vi "Z900_navX_Internal_ProcessingLoop.vi"(11 "navX Device":T2={"Interface"={"Protocol"=enum."SERIAL", "Update Rate (4Hz-100Hz)"=4, "navX Open TypeDef"=variant}, "Notify Packet"=refnum, "Loop VI Refnum"=refnum, "Ready to Close Occurrence Refnum"=refnum} {"Interface"."Update Rate (4Hz-100Hz)" min=4 max=60 step=1}) -> (0 "error out":errorcluster)   [LabVIEW 2015, in "navX Library v2.lvlib"]
doc: "This navX VI handles the reading/writing for the navX. All of the good stuff is in here.\nTHIS VI SHOULD NOT BE CALLED BY THE USER!"
uses:
  navX Library v2.lvlib
  _TypeDefs/Z900_navX_DeviceTypeDef.ctl
  _TypeDefs/Z900_navX_ProtocolTypeDef.ctl
  _TypeDefs/Z900_navX_NotifyPacketTypeDef.ctl
  _TypeDefs/Z900_navX_ActionTypeDef.ctl
  _TypeDefs/Z900_navX_DeviceProcessingLoopStatus.ctl
  <vilib>/Platform/TimedLoop/XDataNode/timing_clust.ctl
  <vilib>/Platform/TimedLoop/XDataNode/nitl_modes.ctl
  <vilib>/Platform/TimedLoop/XDataNode/wakeup.ctl
  _TypeDefs/Z900_navX_InternalTimoutStatusTypeDef.ctl
  SERIAL/Z900_navX_SERIAL_PacketChecksum.vi
  SERIAL/Z900_navX_SERIAL_CapturePacket.vi
  SERIAL/Z900_navX_SERIAL_DecodePacket.vi
  _Util/Decode Protocol/Z900_navX_Util_DecodeProtocol_UInt16.vi
  SERIAL/Z900_navX_SERIAL_ValidatePacketChecksum.vi
  SERIAL/Z900_navX_SERIAL_ValidatePacketTermination.vi
  _Util/Encode Protocol/Z900_navX_Util_EncodeProtocol_SignedHundredths.vi
  _Util/Encode Protocol/Z900_navX_Util_EncodeProtocol_UnsignedHundredths.vi
  _Util/Encode Protocol/Z900_navX_Util_EncodeProtocol_UInt16.vi
  _Util/Z900_navX_Util_LittleEndian_to_BigEndian.vi
  _Util/Encode Protocol/Z900_navX_Util_EncodeProtocol_Int16.vi
  _Util/Z900_navX_Util_BigEndian_to_LittleEndian.vi
  <vilib>/Rock Robotics/WPI/SPI/WPI_SPIClose.vi
  <vilib>/Rock Robotics/WPI/I2C/WPI_I2CClose.vi
  <vilib>/Rock Robotics/WPI/SerialPort/WPI_SerialPortClose.vi
  <vilib>/Rock Robotics/WPI/SerialPort/WPI_SerialPortReset.vi
  <vilib>/Rock Robotics/SystemInterfaces/Utilities/FPGA_UtilitiesRead LocalTime.vi
  <vilib>/Utility/error.llb/Error Cluster From Error Code.vi
  SPI/Z900_navX_SPI_CRC.vi
  <vilib>/Rock Robotics/WPI/SPI/WPI_SPIRead.vi
  <vilib>/Rock Robotics/WPI/SPI/WPI_SPIWrite.vi
  <vilib>/Rock Robotics/WPI/I2C/WPI_I2CRead.vi
  <vilib>/Rock Robotics/WPI/I2C/WPI_I2CWrite.vi
  <vilib>/Rock Robotics/WPI/SerialPort/WPI_SerialPortGetBytesReceived.vi
  <vilib>/Rock Robotics/WPI/SerialPort/WPI_SerialPortRead.vi
  <vilib>/Rock Robotics/WPI/SerialPort/WPI_SerialPortFlush.vi
  <vilib>/Rock Robotics/WPI/SerialPort/WPI_SerialPortWrite.vi
  <vilib>/Rock Robotics/WPI/SPI/WPI_SPIOpen.vi
  <vilib>/Rock Robotics/WPI/I2C/WPI_I2COpen.vi
  <vilib>/Rock Robotics/WPI/SerialPort/WPI_SerialPortTermination.vi
  _NI WPI Serial USB/WPI_SerialPortOpen_USB.vi
  <vilib>/platform/TimedLoop/XDataNode/XDataNode.xnode
  <vilib>/Platform/TimedLoop/XDataNode/XDNodeRunTimeDep.lvlib
panel:
  out "Device ProcessingLoop Status":T1
  in  "Halt":bool
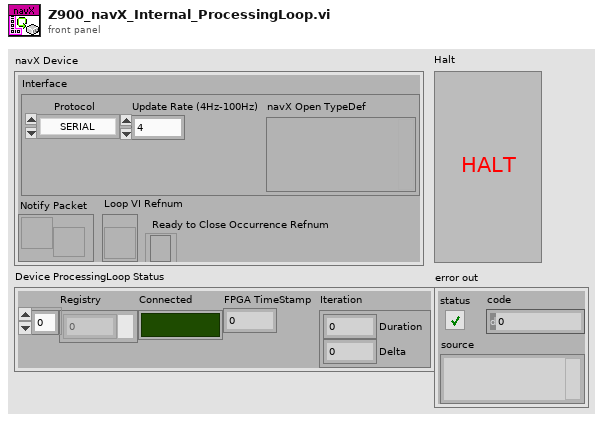
[diagram p1: front panel]
types:
  T1 = typedef "navX Library v2.lvlib/Z900_navX_DeviceProcessingLoopStatus.ctl" = cluster{"Registry":u8[], "Connected":bool, "FPGA TimeStamp":dbl, "Iteration":cluster{"Duration":i64, "Delta":i64}}
  T2 = typedef "navX Library v2.lvlib/Z900_navX_DeviceTypeDef.ctl" = cluster{"Interface":cluster{"Protocol":T3, "Update Rate (4Hz-100Hz)":u8, "navX Open TypeDef":variant}, "Notify Packet":refnum<notifier>, "Loop VI Refnum":refnum<vi>, "Ready to Close Occurrence Refnum":refnum<k4>}
  T3 = typedef "navX Library v2.lvlib/Z900_navX_ProtocolTypeDef.ctl" = enum16{"SERIAL", "I2C", "SPI"}
  T4 = typedef "navX Library v2.lvlib/Z900_navX_InternalTimoutStatusTypeDef.ctl" = cluster{"Last Valid FPGA Time":dbl, "Error Count":i32, "Initialized":bool}
  T5 = typedef "navX Library v2.lvlib/Z900_navX_InterfaceTypeDef.ctl" = cluster{"SerialPortRef":T6, "I2CDevRef":T7, "SPIDevRef":T9}
  T6 = typedef "WPI_SerialPortRef.ctl" = cluster{"DevStatus":errorcluster, "Serial Port Name":refnum<visa-resource-name>}
  T7 = typedef "WPI_I2CDevRef.ctl" = cluster{"DevStatus":errorcluster, "Device Address":u8, "Handle":i32, "I2C Bus":T8}
  T8 = typedef "i2c_bus.ctl" = enum16{"I2C On-Board", "I2C MXP", "Invalid"}
  T9 = typedef "WPI_SPIDevRef.ctl" = cluster{"DevStatus":errorcluster, "Handle":i32, "SPI Bus":T10}
  T10 = typedef "spi_bus.ctl" = enum16{"SPI On-Board, CS0", "SPI On-Board, CS1", "SPI On-Board, CS2", "SPI On-Board, CS3", "SPI MXP", "Invalid"}
  T11 = typedef "XDNodeRunTimeDep.lvlib/timing_clust.ctl" = cluster{"Expected End [f-1]":u64, "Actual End [f-1]":u64, "Finished Late? [f-1]":bool, "Expected End [i-1]":u64, "Actual End [i-1]":u64, "Finished Late? [i-1]":bool, "Expected Start [i]":u64, "Actual Start [i]":u64, "Expected Start [f]":u64, "Actual Start [f]":u64, "Source Name":string, "Structure Name":string, "Period":i64, "Deadline":i64, "Offset":i64, "Start":i64, "Priority":i32, "Timeout":i32, "Mode":T12, "Wakeup Reason":T13, "Error":errorcluster, "Source Type":string, "Secondary Source Type":string, "Global End Time":u64, "Global Start Time":u64, "Frame Duration":u64, "Iteration Duration":u64, "Assigned CPU":i32, "I/O Scan Engine Mode":u32}
  T12 = typedef "XDNodeRunTimeDep.lvlib/nitl_modes.ctl" = enum32{"No Change", "Process missed periods, maintain original phase", "Discard missed periods, maintain original phase", "Process missed periods, ignore original phase", "Discard missed periods, ignore original phase"}
  T13 = typedef "XDNodeRunTimeDep.lvlib/wakeup.ctl" = enum32{"Normal", "Aborted", "Asynchronous wakeup", "Timing source error", "Timed loop error", "Timeout"}
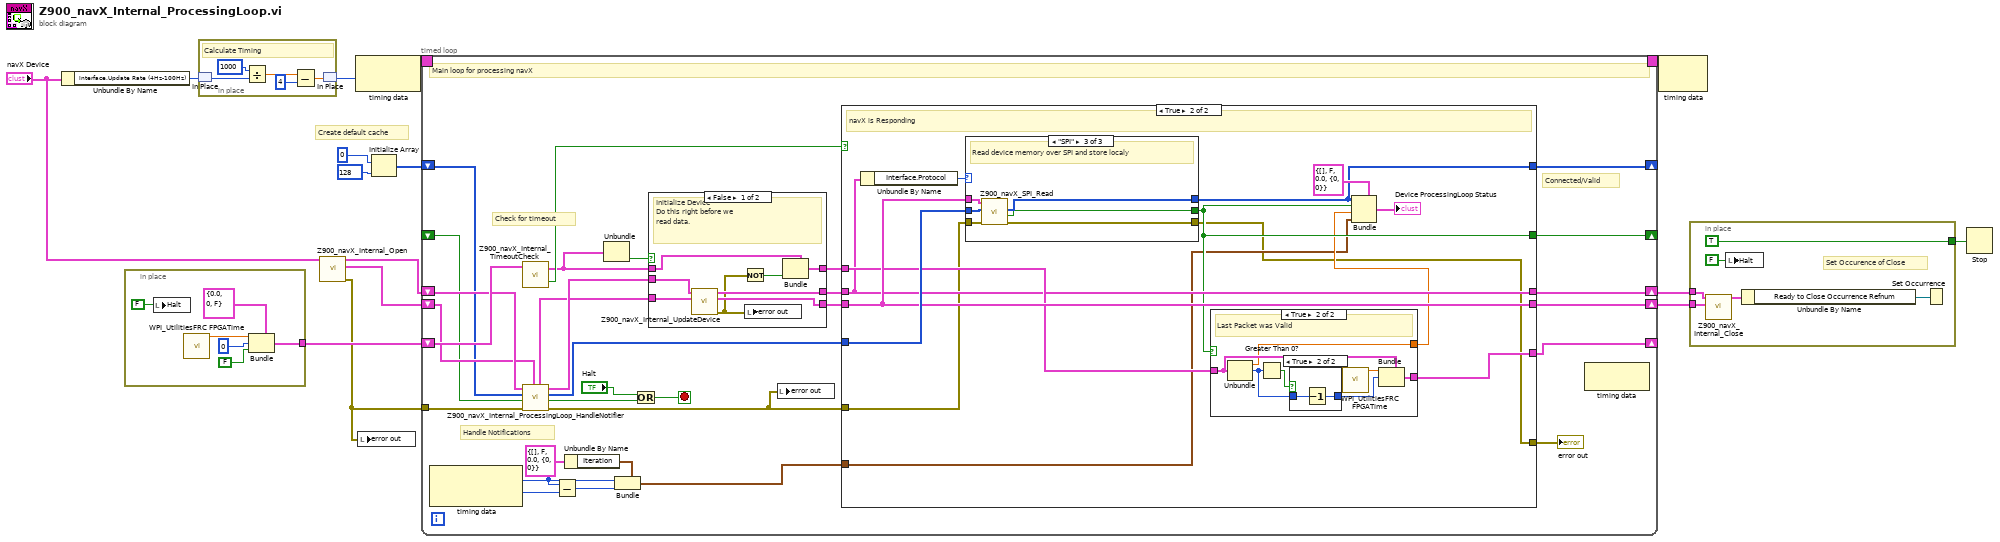
[diagram p0: block diagram]
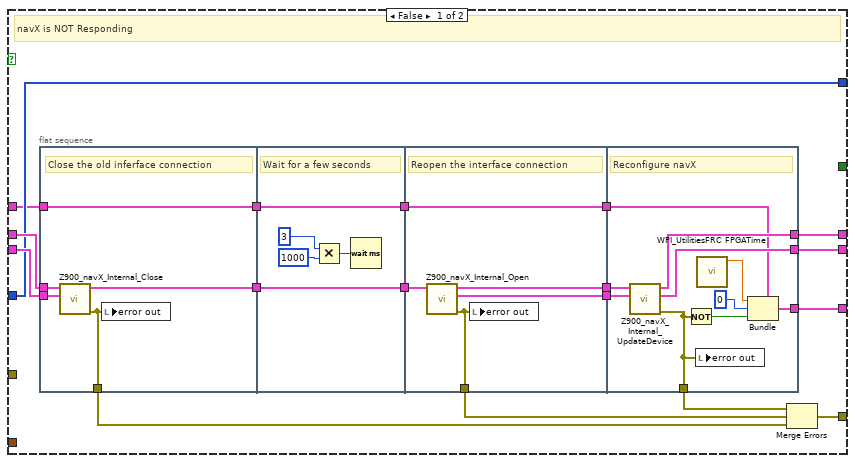
[diagram p3: hidden frame]
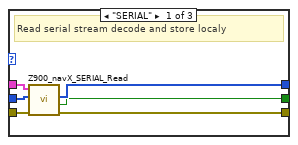
[diagram p4: hidden frame]
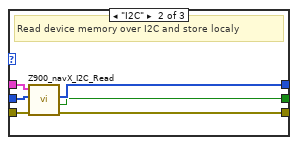
[diagram p5: hidden frame]
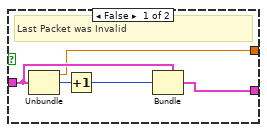
[diagram p6: hidden frame]
diagram:
  # "Create default cache"
  n1 = Unbundle By Name("navX Device") -> ("Interface.Update Rate (4Hz-100Hz)"=w12:u8)
  n2 = in-place {
    in-place-border: [w19] -> w7
    n3 = local write "Halt"(FALSE ("Halt")) -> ()
    n4 = call <vilib>:"WPI_UtilitiesFRC FPGATime.vi"() -> ("FPGA Time"=w20:dbl)  [unwired: 10 in, 1 out]
    n5 = Bundle(cluster=T4 {"Last Valid FPGA Time"=0.0, "Error Count"=0, "Initialized"=FALSE}, "Last Valid FPGA Time"=w20, "Error Count"=0, "Initialized"=FALSE) -> (w19:T4)
  }
  n6 = in-place {
    # "Calculate Timing"
    n7 = in-place-match #1(w12) -> (w25:u8)
    n8 = Divide(x=1000, y=w25) -> (x/y=w23:dbl)
    n9 = Subtract(x=w23, y=4) -> (x-y=w22:dbl)
    n10 = in-place-match #1(w22) -> (w13:u8)
  }
  n11 = call "Z900_navX_Internal_Open.vi"("navX Device"="navX Device") -> ("error out"=w1:errorcluster, "Interface TypeDefs"=w8:T5, "navX Device"=w6:T2)  [unwired: 8 in]
  n12 = node-c288(w13) -> (w15:T11)
  n13 = local write "error out"(w1) -> ()
  n14 = Initialize Array(u8 0 ("Received Data"), 128 ("hex")) -> (w11:u8[])
  n15 = timed-loop {
    timing: w15 -> [_]
    timing-out: [_] -> w14
    shift-right: [w57] -> _
    shift-left: w11 -> [w43]
    shift-right: [w54] -> w10
    shift-left: w6 -> [w45]
    shift-right: [w55] -> w9
    shift-left: w8 -> [w44]
    shift-right: [w56] -> _
    shift-left: w7 -> [w49]
    tunnel: w1 -> [w41]
    shift-right: [w46] -> _
    shift-left: _ -> [w42]
    stop <- w34 stop-if-true
    # "Check for timeout"
    # "Handle Notifications"
    # "Connected/Valid"
    # "Main loop for processing navX"
    n16 = node-c288() -> (w29:i64, w33:i64)  [unwired: 1 in]
    n17 = call "Z900_navX_Internal_TimeoutCheck.vi"("Timout Status (in)"=w49) -> ("TIMEOUT!"=w48:bool, "Timout Status (out)"=w47:T4)  [unwired: 2 in]
    n18 = call "Z900_navX_Internal_ProcessingLoop_HandleNotifier.vi"("Interface TypeDefs"=w44, "error in (no error)"=w41, "Connected"=w42, "Registry"=w43, "navX Device"=w45) -> ("error out"=w37:errorcluster, "Halt"=w36:bool, "Registry"=w38:u8[], "navX Device"=w40:T2, "Interface TypeDefs"=w39:T5)  [unwired: 2 in]
    n19 = Subtract(x=w29, y=w33) -> (x-y=w28:i64)
    n20 = Unbundle By Name(T1 {"Registry"=[], "Connected"=FALSE, "FPGA TimeStamp"=0.0, "Iteration"={"Duration"=0, "Delta"=0}} ("Device ProcessingLoop Status")) -> ("Iteration"=w30:cluster{"Duration":i64, "Delta":i64})
    n21 = Unbundle(w47) -> ("Initialized"=w53:bool)  [unwired: 2 out]
    n22 = Bundle(cluster=w30, "Duration"=w29, "Delta"=w28) -> (w27:cluster{"Duration":i64, "Delta":i64})
    n23 = Or(x="Halt", y=w36) -> (x .or. y?=w34:bool)
    n24 = case shown="False" w53 {
      tunnel: w47 -> [w65 w68]
      tunnel: [w64 w68] -> w52
      tunnel: w40 -> [w63 w67]
      tunnel: w39 -> [w62 w66]
      tunnel: [w61 w67] -> w50
      tunnel: [w60 w66] -> w51
      frame False {
        # "Initialize Device\nDo this right before we\nread data."
        n25 = call "Z900_navX_Internal_UpdateDevice.vi"("Interface TypeDefs"=w62, "navX Device"=w63) -> ("error out"=w59:errorcluster, "Interface TypeDefs"=w60:T5, "navX Device"=w61:T2)  [unwired: 7 in]
        n26 = Not(x=w59) -> (.not. x?=w58:bool)
        n27 = local write "error out"(w59) -> ()
        n28 = Bundle(cluster=w65, "Initialized"=w58) -> (w64:T4)  [unwired: 2 in]
      }
      frame True {
      }
    }
    n29 = local write "error out"(w37) -> ()
    n30 = case shown="True" w48 {
      tunnel: w38 -> [w84 w125]
      tunnel: w51 -> [w85 w124]
      tunnel: [w84 w119] -> w57
      tunnel: w52 -> [w73 w123]
      tunnel: [w77 w122] -> w56
      tunnel: w50 -> [w86 w121]
      tunnel: [w78 w121] -> w54
      tunnel: [w81 w124] -> w55
      tunnel: w37 -> [_ w118]
      tunnel: [_ w117] -> w46
      tunnel: [w69 w112] -> w32
      tunnel: w27 -> [_ w113]
      frame False {
        # "navX is NOT Responding"
        n31 = flat-sequence {
          tunnel: w86 -> [w89]
          tunnel: w85 -> [w91]
          tunnel: [w90] -> w83
          tunnel: [w88] -> w74
          tunnel: w73 -> [w88]
          tunnel: [w87] -> w70
          tunnel: w83 -> [w96]
          tunnel: [w96] -> w82
          tunnel: [w92] -> w75
          tunnel: w74 -> [w92]
          tunnel: w82 -> [w100]
          tunnel: [w101] -> w80
          tunnel: [w99] -> w79
          tunnel: [w98] -> w76
          tunnel: w75 -> [w98]
          tunnel: [w97] -> w71
          tunnel: [w110] -> w77
          tunnel: [w106] -> w81
          tunnel: [w107] -> w78
          tunnel: w76 -> [w105]
          tunnel: w79 -> [w108]
          tunnel: w80 -> [w109]
          tunnel: [w102] -> w72
          frame #0 {
            # "Close the old inferface connection"
            n32 = call "Z900_navX_Internal_Close.vi"("Interface TypeDefs"=w91, "navX Device"=w89) -> ("error out"=w87:errorcluster, "navX Device"=w90:T2)  [unwired: 8 in]
            n33 = local write "error out"(w87) -> ()
          }
          frame #1 {
            # "Wait for a few seconds"
            n34 = Multiply(x=u32 3 ("milliseconds to wait"), y=u32 1000) -> (x*y=w94:u32)
            n35 = Wait (ms)(milliseconds to wait=w94) -> ()  [unwired: 1 out]
          }
          frame #2 {
            # "Reopen the interface connection"
            n36 = call "Z900_navX_Internal_Open.vi"("navX Device"=w100) -> ("error out"=w97:errorcluster, "Interface TypeDefs"=w99:T5, "navX Device"=w101:T2)  [unwired: 8 in]
            n37 = local write "error out"(w97) -> ()
          }
          frame #3 {
            # "Reconfigure navX"
            n38 = call "Z900_navX_Internal_UpdateDevice.vi"("Interface TypeDefs"=w108, "navX Device"=w109) -> ("error out"=w102:errorcluster, "Interface TypeDefs"=w106:T5, "navX Device"=w107:T2)  [unwired: 7 in]
            n39 = Not(x=w102) -> (.not. x?=w111:bool)
            n40 = local write "error out"(w102) -> ()
            n41 = call <vilib>:"WPI_UtilitiesFRC FPGATime.vi"() -> ("FPGA Time"=w104:dbl)  [unwired: 10 in, 1 out]
            n42 = Bundle(cluster=w105, "Last Valid FPGA Time"=w104, "Error Count"=0, "Initialized"=w111) -> (w110:T4)
          }
        }
        n43 = Merge Errors(w72, w71, w70) -> (w69:errorcluster)
      }
      frame True {
        # "navX is Responding"
        n44 = Unbundle By Name(w121) -> ("Interface.Protocol"=w116:T3)
        n45 = case shown="\"SPI\"" w116 {
          tunnel: [w127 w135 w141] -> w119
          tunnel: w125 -> [w130 w136 w142]
          tunnel: w124 -> [w131 w137 w143]
          tunnel: [w126 w134 w140] -> w117
          tunnel: w118 -> [w129 w133 w139]
          tunnel: [w128 w132 w138] -> w112
          frame "SERIAL" {
            # "Read serial stream decode and store localy"
            n46 = call "Z900_navX_SERIAL_Read.vi"("error in (no error)"=w129, "Registry"=w130, "Interface TypeDefs"=w131) -> ("error out"=w128:errorcluster, "Valid"=w126:bool, "Registry"=w127:u8[])  [unwired: 5 in, 1 out]
          }
          frame "I2C" {
            # "Read device memory over I2C and store localy"
            n47 = call "Z900_navX_I2C_Read.vi"("error in (no error)"=w133, "Registry"=w136, "Interface TypeDefs"=w137) -> ("error out"=w132:errorcluster, "Valid"=w134:bool, "Registry"=w135:u8[])  [unwired: 5 in, 1 out]
          }
          frame "SPI" {
            # "Read device memory over SPI and store localy"
            n48 = call "Z900_navX_SPI_Read.vi"("error in (no error)"=w139, "Registry"=w142, "Interface TypeDefs"=w143) -> ("error out"=w138:errorcluster, "Valid"=w140:bool, "Registry"=w141:u8[])  [unwired: 5 in, 1 out]
          }
        }
        n49 = case shown="True" w117 {
          tunnel: [w145 w154] -> w122
          tunnel: w123 -> [w146 w153]
          tunnel: [w144 w149] -> w114
          frame False {
            # "Last Packet was Invalid"
            n50 = Unbundle(w146) -> ("Last Valid FPGA Time"=w144:dbl, "Error Count"=w147:i32)  [unwired: 1 out]
            n51 = Increment(x=w147) -> (x+1=w148:i32)
            n52 = Bundle(cluster=w146, "Error Count"=w148) -> (w145:T4)  [unwired: 2 in]
          }
          frame True {
            # "Last Packet was Valid"
            n53 = Unbundle(w153) -> ("Last Valid FPGA Time"=w149:dbl, "Error Count"=w151:i32)  [unwired: 1 out]
            n54 = Greater Than 0?(x=w151) -> (x > 0?=w152:bool)
            n55 = case shown="True" w152 {
              tunnel: [w156 w157] -> w150
              tunnel: w151 -> [w156 w158]
              frame False {
              }
              frame True {
                n56 = Decrement(x=w158) -> (x-1=w157:i32)
              }
            }
            n57 = call <vilib>:"WPI_UtilitiesFRC FPGATime.vi"() -> ("FPGA Time"=w155:dbl)  [unwired: 10 in, 1 out]
            n58 = Bundle(cluster=w153, "Last Valid FPGA Time"=w155, "Error Count"=w150) -> (w154:T4)  [unwired: 1 in]
          }
        }
        n59 = Bundle(cluster=T1 {"Registry"=[], "Connected"=FALSE, "FPGA TimeStamp"=0.0, "Iteration"={"Duration"=0, "Delta"=0}} ("Device ProcessingLoop Status"), "Registry"=w119, "Connected"=w117, "FPGA TimeStamp"=w114, "Iteration"=w113) -> (→"Device ProcessingLoop Status":T1)
      }
    }
    "error out" <- w32
    n60 = node-c288() -> ()  [unwired: 1 in, 1 out]
  }
  n61 = node-c288(w14) -> ()  [unwired: 1 out]
  n62 = in-place {
    in-place-border: w10 -> [w168]
    in-place-border: w9 -> [w167]
    in-place-border: [TRUE] -> w5
    # "Set Occurence of Close"
    n63 = call "Z900_navX_Internal_Close.vi"("Interface TypeDefs"=w167, "navX Device"=w168) -> ("navX Device"=w163:T2)  [unwired: 8 in, 1 out]
    n64 = local write "Halt"(FALSE ("Halt")) -> ()
    n65 = Unbundle By Name(w163) -> ("Ready to Close Occurrence Refnum"=w165:refnum<k4>)
    n66 = Set Occurrence(w165) -> ()
  }
  n67 = Stop(stop? (T)=w5) -> ()
